vi "Notifier References FGV.vi"(8 "error in":errorcluster, 11 "function":enum16{"obtain", "get", "release"}(ring)) -> (0 "error out":errorcluster, 3 "module notifiers":T1)   [LabVIEW 2017, in "Logger.lvlib"]
uses:
  Logger.lvlib
  Private TypeDefs/Module Notifiers.ctl
  Private TypeDefs/Dummy Notifier.ctl
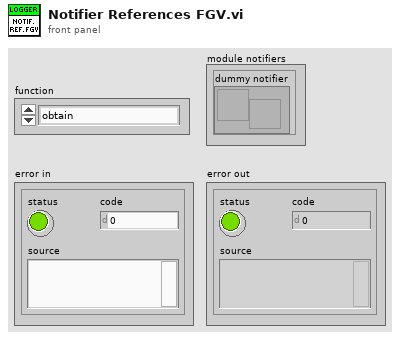
[diagram p1: front panel]
types:
  T1 = typedef "Logger.lvlib/Module Notifiers.ctl" = cluster{"dummy notifier":refnum<notifier>}
  T2 = typedef "Logger.lvlib/Dummy Notifier.ctl" = cluster{"Numeric":dbl}
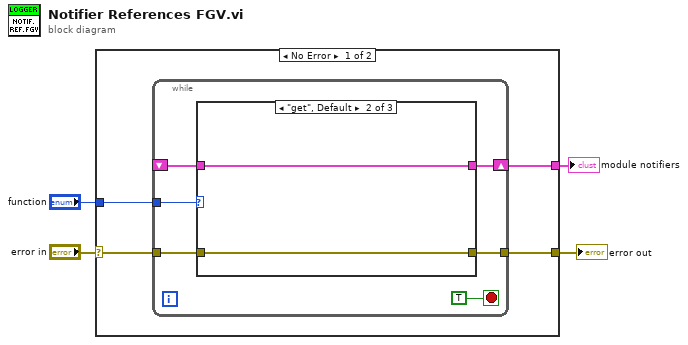
[diagram p0: block diagram]
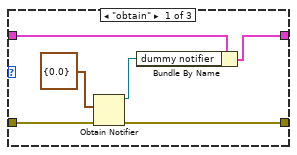
[diagram p2: hidden frame]
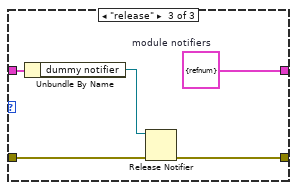
[diagram p3: hidden frame]
diagram:
  n1 = case shown="No Error" "error in" {
    selector: "error in" -> [w8 w28]
    tunnel: [w7 w28] -> w3
    tunnel: "function" -> [w6 _]
    tunnel: [w5 _] -> w1
    frame No Error {
      n2 = while {
        tunnel: w8 -> [w13]
        tunnel: [w12] -> w7
        tunnel: w6 -> [w11]
        shift-right: [w10] -> w5
        shift-left: _ -> [w9]
        stop <- TRUE stop-if-true
        n3 = case shown="\"get\", Default" w11 {
          tunnel: w13 -> [w20 w22 w27]
          tunnel: [w19 w22 w26] -> w12
          tunnel: [w17 w21 w25] -> w10
          tunnel: w9 -> [w18 w21 w24]
          frame "obtain" {
            n4 = Obtain Notifier(notification data type=T2 {"Numeric"=0.0}, error in (no error)=w20) -> (notifier out=w15:refnum<notifier>, error out=w19:errorcluster)  [unwired: 2 in, 1 out]
            n5 = Bundle By Name(cluster=w18, "dummy notifier"=w15) -> (w17:T1)
          }
          frame "get", Default {
          }
          frame "release" {
            w25 = T1 {"dummy notifier"=refnum}  # module notifiers
            n6 = Unbundle By Name(w24) -> ("dummy notifier"=w23:refnum<notifier>)
            n7 = Release Notifier(notifier=w23, error in (no error)=w27) -> (error out=w26:errorcluster)  [unwired: 1 in, 2 out]
          }
        }
      }
    }
    frame Error {
    }
  }
  "error out" <- w3
  "module notifiers" <- w1
